vi "Actor.vi"(11 "Polled_EventSource":refnum<class "Polled_EventSource.lvclass">) -> ()   [LabVIEW 2021, in "Polled_EventSource.lvclass"]
uses:
  Polled_EventSource.lvclass
  Polled_EventSource.lvclass/Polled_EventSource.ctl
  <vilib>/platform/TimedLoop/XDataNode/XDataNode.xnode
  <vilib>/Platform/TimedLoop/XDataNode/nitl_modes.ctl
  <vilib>/Platform/TimedLoop/XDataNode/XDNodeRunTimeDep.lvlib
  <vilib>/Platform/TimedLoop/XDataNode/wakeup.ctl
  <vilib>/Platform/TimedLoop/XDataNode/timing_clust.ctl
  Event_Polled Type.lvclass
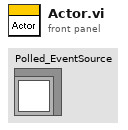
[diagram p1: front panel]
types:
  T1 = typedef "XDNodeRunTimeDep.lvlib/timing_clust.ctl" = cluster{"Expected End [f-1]":u64, "Actual End [f-1]":u64, "Finished Late? [f-1]":bool, "Expected End [i-1]":u64, "Actual End [i-1]":u64, "Finished Late? [i-1]":bool, "Expected Start [i]":u64, "Actual Start [i]":u64, "Expected Start [f]":u64, "Actual Start [f]":u64, "Source Name":string, "Structure Name":string, "Period":i64, "Deadline":i64, "Offset":i64, "Start":i64, "Priority":i32, "Timeout":i32, "Mode":T2, "Wakeup Reason":T3, "Error":errorcluster, "Source Type":string, "Secondary Source Type":string, "Global End Time":u64, "Global Start Time":u64, "Frame Duration":u64, "Iteration Duration":u64, "Assigned CPU":i32, "I/O Scan Engine Mode":u32}
  T2 = typedef "XDNodeRunTimeDep.lvlib/nitl_modes.ctl" = enum32{"No Change", "Process missed periods, maintain original phase", "Discard missed periods, maintain original phase", "Process missed periods, ignore original phase", "Discard missed periods, ignore original phase"}
  T3 = typedef "XDNodeRunTimeDep.lvlib/wakeup.ctl" = enum32{"Normal", "Aborted", "Asynchronous wakeup", "Timing source error", "Timed loop error", "Timeout"}
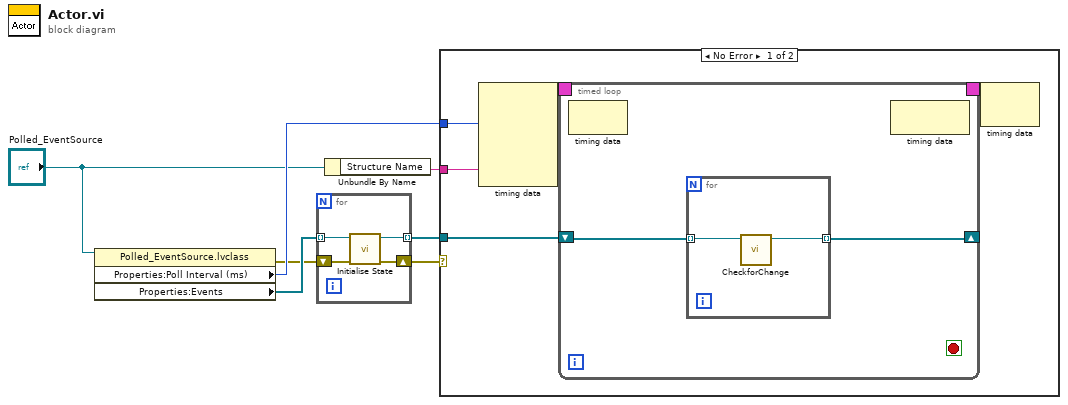
[diagram p0: block diagram]
diagram:
  n1 = property class="Polled_EventSource.lvclass"(reference="Polled_EventSource") -> (error out=w1:errorcluster, "Properties:Poll Interval (ms)"=w7:i32, "Properties:Events"=w4:refnum<class "Event_Polled Type.lvclass">[])  [unwired: 1 in, 1 out]
  n2 = for {
    tunnel: w4 -> [w11] mode=indexing
    tunnel: [w10] -> w3 mode=indexing
    shift-right: [w8] -> w2
    shift-left: w1 -> [w9]
    n3 = call-dynamic "Initialise State.vi"("error in (no error)"=w9, "Event_Polled Type.lvclass in"=w11) -> ("error out"=w8:errorcluster, "Event_Polled Type.lvclass out"=w10:refnum<class "Event_Polled Type.lvclass">)  [unwired: 8 in]
  }
  n4 = Unbundle By Name("Polled_EventSource") -> ("Structure Name"=w6:string)
  n5 = case shown="No Error" w2 {
    tunnel: w7 -> [w14 _]
    tunnel: w6 -> [w13 _]
    tunnel: w3 -> [w12 _]
    frame No Error {
      n6 = node-c288(w14, w13) -> (w16:T1)  [unwired: 3 in]
      n7 = timed-loop {
        timing: w16 -> [_]
        timing-out: [_] -> w15
        shift-right: [w18] -> _
        shift-left: w12 -> [w17]
        stop <- _ stop-if-true
        n8 = node-c288() -> ()  [unwired: 1 in, 1 out]
        n9 = for {
          tunnel: [w19] -> w18 mode=indexing
          tunnel: w17 -> [w20] mode=indexing
          n10 = call-dynamic "CheckforChange.vi"("Event_Polled Type.lvclass in"=w20) -> ("Event_Polled Type.lvclass out"=w19:refnum<class "Event_Polled Type.lvclass">)  [unwired: 9 in, 1 out]
        }
        n11 = node-c288() -> ()  [unwired: 1 in, 1 out]
      }
      n12 = node-c288(w15) -> ()  [unwired: 1 out]
    }
    frame Error {
    }
  }
